vi "Sent Get Joystick State WFR.vi"(7 "Message Priority (Normal)":T2=enum."Normal", 8 "error in (no error)":errorcluster, 11 "Message Enqueuer":refnum<class "Message Enqueuer.lvclass">) -> (0 "error out":errorcluster, 2 "Reply":T1, 3 "Message Enqueuer out":refnum<class "Message Enqueuer.lvclass">)   [LabVIEW 2020, in "RPI.SenseHat.Actor.lvlib" / "Get Joystick State Msg WFR.lvclass"]
uses:
  <vilib>/ActorFramework/Message Enqueuer/Message Enqueuer.lvclass
  <vilib>/ActorFramework/Message Enqueuer/Message Priority.ctl
  RPI.SenseHat.Joystick/TypeDefs/Joystick.ctl
  Get Joystick State Msg WFR.lvclass
  C:/Program Files (x86)/National Instruments/LabVIEW 2020/vi.lib/ActorFramework/Reply Msg/Reply Msg.lvclass
  <vilib>/ActorFramework/Reply Msg/Reply Msg.lvclass/Reply Msg.ctl
  <vilib>/ActorFramework/Message Enqueuer/Message Enqueuer.lvclass/Message Enqueuer.ctl
  <vilib>/ActorFramework/Message Enqueuer/Enqueue.vi
  <vilib>/ActorFramework/Reply Msg/Reply Msg.lvclass
  C:/Program Files (x86)/National Instruments/LabVIEW 2020/vi.lib/ActorFramework/Message/Message.lvclass
  <vilib>/ActorFramework/Message Priority Queue/Priority Enqueue.vi
  RPI.SenseHat.Joystick/RPI.SenseHat.Joystick.lvlib
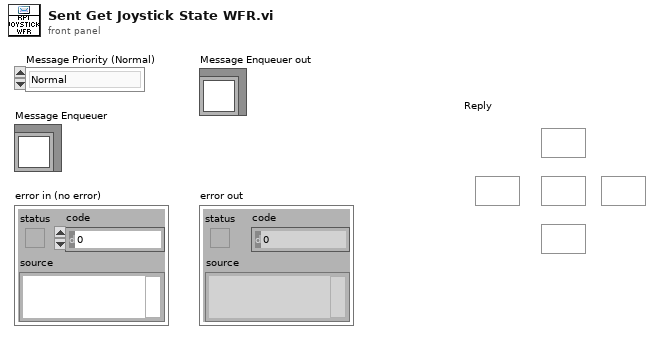
[diagram p1: front panel]
types:
  T1 = typedef "RPI.SenseHat.Joystick.lvlib/Joystick.ctl" = cluster{"Enter":bool, "Down":bool, "Up":bool, "Right":bool, "Left":bool}
  T2 = typedef "Actor Framework.lvlib/Message Enqueuer.lvclass/Message Priority.ctl" = enum16{"Low", "Normal", "High"}
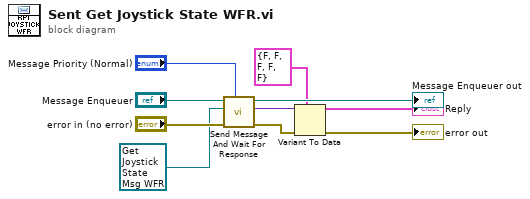
[diagram p0: block diagram]
diagram:
  n1 = call <vilib>:"Send Message And Wait For Response.vi"("Message Priority (Normal)"="Message Priority (Normal)", "error in (no error)"="error in (no error)", "Original Message"=refnum<class "Get Joystick State Msg WFR.lvclass"> refnum ("RPI.SenseHat.Actor.lvlib:Get Joystick State Msg WFR.lvclass"), "Message Enqueuer in"="Message Enqueuer") -> ("error out"=w5:errorcluster, "Reply"=w6:variant, "Message Enqueuer out"=→"Message Enqueuer out":refnum<class "Message Enqueuer.lvclass">)  [unwired: 4 in, 1 out]
  n2 = Variant To Data(error in=w5, type=T1 {"Enter"=FALSE, "Down"=FALSE, "Up"=FALSE, "Right"=FALSE, "Left"=FALSE} ("Joystick"), Variant=w6) -> (data=→"Reply":T1, error out=→"error out":errorcluster)
